vi "ScriptBreakout.vi"(11 "Script":string) -> (0 "Rest":string, 1 "Commands":string[](array[string]), 2 "VI Name":string[](array[string]), 3 "Padding":string[](array[string]))   [LabVIEW 2021, in "ScriptManager.lvlib"]
uses:
  <vilib>/regexp/Match Regular Expression.xnode
  ScriptManager.lvlib
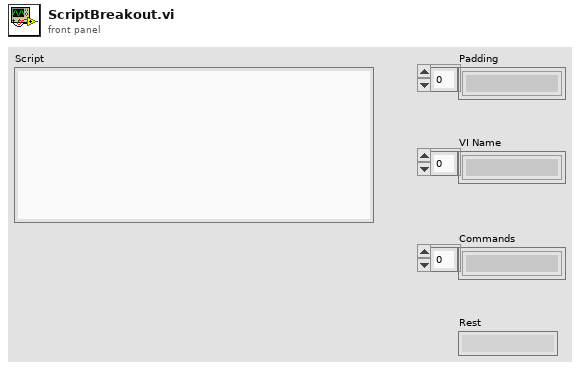
[diagram p1: front panel]
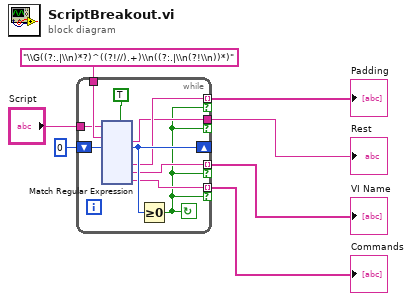
[diagram p0: block diagram]
diagram:
  n1 = while {
    tunnel: "Script" -> [w16]
    tunnel: "\\G((?:.|\\n)*?)^((?!//).+)\\n((?:.|\\n(?!\\n))*)" ("regular expression") -> [w17]
    tunnel: [w10] -> w6 mode=indexing if=w8
    tunnel: [w9] -> w7 if=w8
    tunnel: [w11] -> w5 mode=indexing if=w8
    tunnel: [w12] -> w4 mode=indexing if=w8
    shift-right: [w14] -> _
    shift-left: 0 -> [w15]
    stop <- w8 continue-if-true
    n2 = xnode "Match Regular Expression"("input string"=w16, "regular expression"=w17, "offset (0)"=w15, "multiline? (F)"=TRUE) -> ("after match"=w9:string, "offset past match"=w14:i32, "submatch 1"=w10:string, "submatch 2"=w11:string, "submatch 3"=w12:string)  [unwired: 2 in, 3 out]
    n3 = Greater Or Equal To 0?(x=w14) -> (x >= 0?=w8:bool)
  }
  "Rest" <- w7
  "Padding" <- w6
  "VI Name" <- w5
  "Commands" <- w4
